vi "MPM_Sample.vi"() -> ()   [LabVIEW 2017]
uses:
  C:/Users/Ssantec_Test/Documents/Instrument_DLL_Sample_Labview_20250826_Ver1.5.0_x64/DLL/InstrumentDLL.dll
  DLL/InstrumentDLL.dll
  <vilib>/Utility/file.llb/Write Delimited Spreadsheet (string).vi
  <vilib>/Utility/file.llb/Write To Spreadsheet File (DBL).vi
panel:
  out "MPM":refnum<k24>
  in  "选项卡控件":T1(tab)
  out "lblver4":string
  out "lblseri4":string
  out "lbltype4":string
  out "lblver3":string
  out "lblseri3":string
  out "lbltype3":string
  out "lblver2":string
  out "lblseri2":string
  out "lbltype2":string
  out "lblver1":string
  out "lblseri1":string
  out "lbltype1":string
  out "lblver0":string
  out "lblseri0":string
  out "lbltype0":string
  out "module count":string
  out "Product":string
  out "Serial":string
  out "F/ W Vesion":string
  in  "btnDisconnect":bool
  in  "btnConnect":bool
  in  "Portnumber":i32
  in  "Address/ComPort":string
  in  "Communication":T2(radio)
  in  "GetComport":bool
  in  "ComPort":u16(ring)
  in  "btnSplit":bool
  out "Address":dbl
  out "Board number":dbl
  in  "btnVisa":bool
  in  "Visa String":u16(ring) items=["GPIB0::16::INSTR"]
  out "txtlan_port":string
  in  "btnGetPort":bool
  out "txtipaddress":string
  in  "btnGetIP":bool
  out "txtsyst_error":string
  in  "btnGetError":bool
  in  "btnGetWavelength":bool
  in  "txtwave_ch":i32 caption="Ch"
  in  "txtwave_slot":i32 caption="Slot"
  in  "btnZeroing":bool
  out "txtreadp_all":string caption="Read Power for each slot"
  in  "txtread_slotall":i32 caption="Slot"
  in  "btnSlot_Power":bool
  out "txt_readp_ch":dbl caption="Read Power for each ch"
  in  "txtread_ch":i32=1 caption="Ch"
  in  "txtread_slot":i32 caption="Slot"
  in  "btnSlot_Ch_Power":bool
  out "txtget_erange":dbl caption="Range for each ch"
  in  "txtget_rangech":i32=1 caption="Ch"
  in  "txtget_rangeslot":i32 caption="Slot"
  out "txtgetrmode":string caption="Range mode for \"READ\""
  in  "btnSlot_Ch_Range":bool
  in  "btnGet":bool
  out "txtget_unit":string caption="Unit"
  out "txtget_avg":dbl caption="Averaging time(msec)"
  out "txtget_wave":dbl caption="Wavelength(nm)"
  out "txtgetrang":i32 caption="Range All"
  in  "Ch":i32
  in  "Slot":i32
  in  "Range for each ch":i32
  in  "btnSetSlot":bool
  in  "Averaging time(msec)":dbl
  in  "btnSetAveraging":bool
  in  "btnSetUnit":bool
  in  "Unit":u16(ring) items=["dBm", "mW"]
  in  "btnSetRangeAll":bool
  in  "Range All":i32
  in  "btnSetRangeMode":bool
  in  "Range mode for \"READ\"":enum16{"Auto", "Manual"}(ring)
  in  "Wavelength(nm)":dbl
  in  "btnSetWavelength":bool
  in  "btnGetSlot":bool
  in  "txte_slot":i32 caption="Slot"
  in  "btnGetch":bool
  in  "txtlog_ch":i32 caption="Ch"
  in  "txtlog_slot":i32 caption="Slot"
  out "txtlog_status":string
  in  "btnStop":bool
  in  "btnStatus":bool
  in  "btnStart":bool
  in  "btnSetFreerun":bool
  in  "cmbfr_tin_mode":enum16{"Internal", "Extarnal"}(ring) caption="Trigger input mode"
  in  "txtfr_range":i32 caption="Range"
  in  "txtfr_point":i32 caption="number of point"
  in  "txtfr_ave":dbl caption="Averaging Time(msec)"
  in  "txtfr_wave":dbl caption="Wavelength(nm)"
  in  "btnSetSweep":bool
  in  "txtsm_range":i32 caption="Range"
  in  "cmbsm_rangemode":enum16{"Auto", "Manual"}(ring) caption="Range mode"
  in  "txtspeed":i32 caption="Speed(nm/sec)"
  in  "txtwavestep":dbl caption="Step wavelenght(nm)"
  in  "txtstopwave":dbl caption="Stop wavelenght(nm)"
  in  "txtstartwave":dbl caption="Start wavelength(nm)"
  in  "txtcon_range":i32 caption="Range"
  in  "cmbcon_rangemode":enum16{"Auto", "Manual"}(ring) caption="Range mode"
  in  "txtcon_point":i32 caption="number of point"
  in  "txtcon_ave":dbl caption="Averaging Time(msec)"
  in  "txtcon_wave":dbl caption="Wavelength(nm)"
  in  "btnSetConst":bool
  in  "btnGetParameter":bool
  out "txtg_speed":dbl caption="Sweep speed(nm)"
  out "txtg_stepwave":dbl caption="Step wavelength(nm)"
  out "txtg_stopwave":dbl caption="Stop wavelength(nm)"
  out "txtg_statwave":dbl caption="Start wavelength(nm)"
  out "txtg_wavelength":dbl caption="Wavelength(nm)"
  out "txtg_settingrange":string caption="Setting Range"
  out "txtg_tinmode":string caption="Trigger input mode"
  out "txtg_rangemode":string caption="Range mode"
  out "txtlog_mode":string caption="SweepMode"
  out "txtg_point":i32 caption="number of point"
  out "txtg_ave":dbl caption="Averaging time"
  # "0. Connect Tool"
  # "1. Connect"
  # "Communication setting"
  # "Information"
  # "Module Information"
  # "Slot0"
  # "Slot1"
  # "Slot2"
  # "Slot3"
  # "Slot4"
  # "Type"
  # "Serial"
  # "Version"
  # "Set"
  # "Get"
  # "Common function"
  # "Const Mode"
  # "Sweep Mode"
  # "FreerunMode"
  # "Common"
  # "Get Parameter"
  # "Sweep mode parameter"
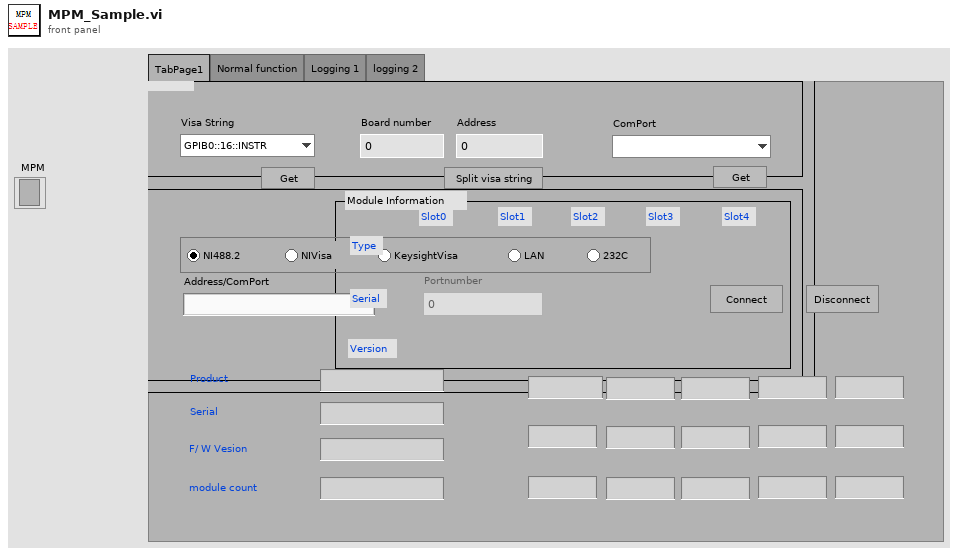
[diagram p1: front panel]
types:
  T1 = enum32{"TabPage1", "Normal function", "Logging 1", "logging 2"}
  T2 = enum32{"rdiNI488", "rdiNIvisa", "rdikeysightvisa", "rdiLAN", "rdi232C"}
  T3 = enum8{"Enabled", "Disabled", "Disabled and Grayed Out"}
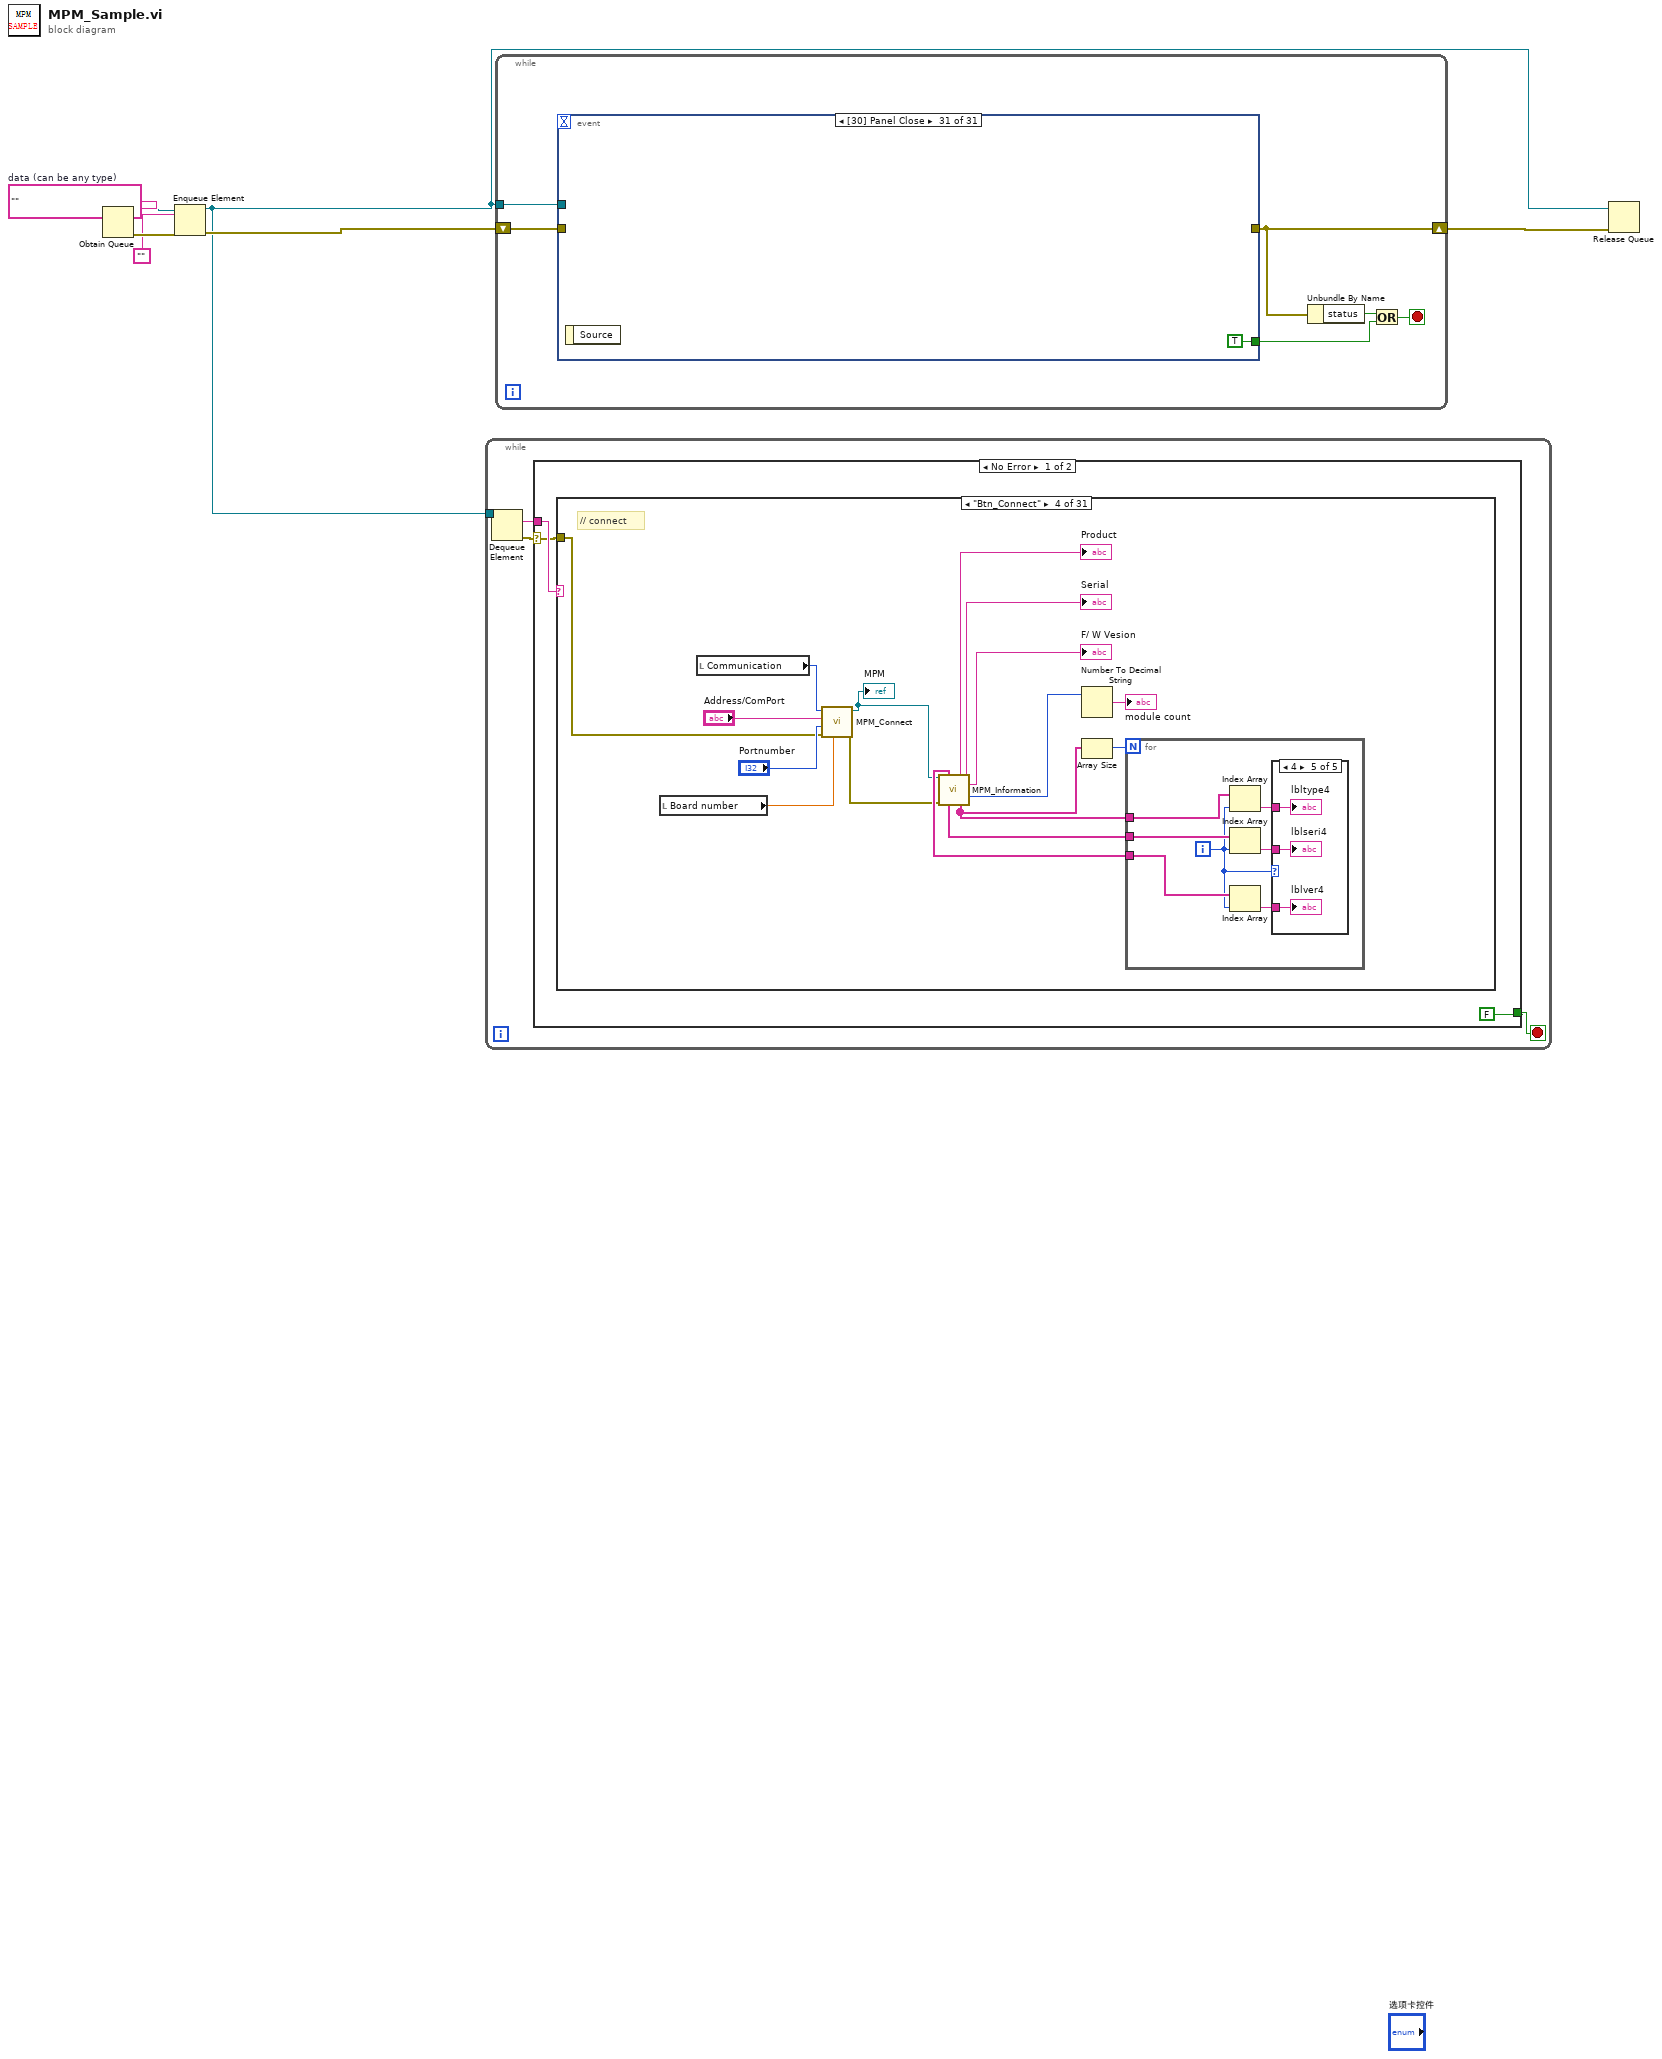
[diagram p0: block diagram]
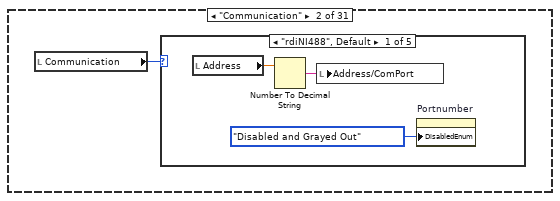
[diagram p3: hidden frame]
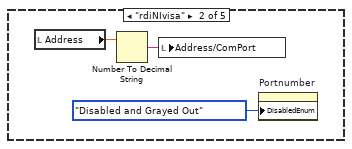
[diagram p4: hidden frame]
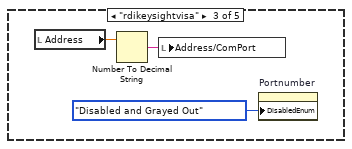
[diagram p5: hidden frame]
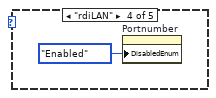
[diagram p6: hidden frame]
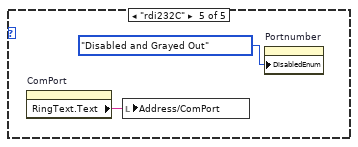
[diagram p7: hidden frame]
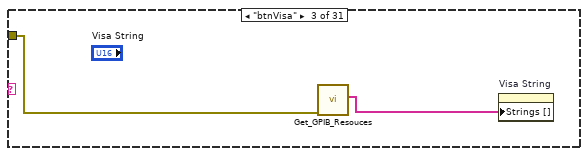
[diagram p8: hidden frame]
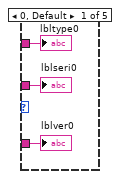
[diagram p9: hidden frame]
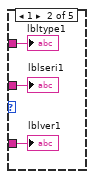
[diagram p10: hidden frame]
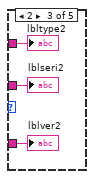
[diagram p11: hidden frame]
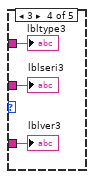
[diagram p12: hidden frame]
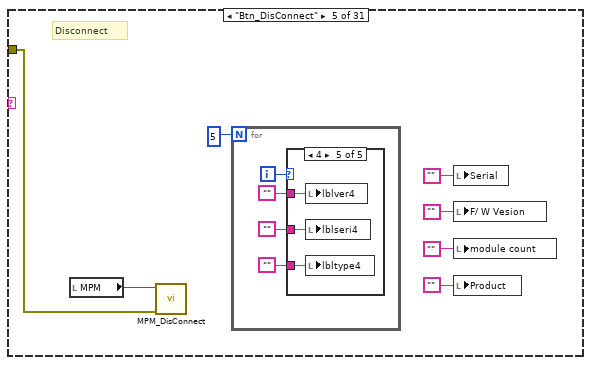
[diagram p13: hidden frame]
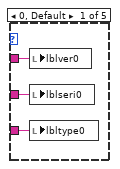
[diagram p14: hidden frame]
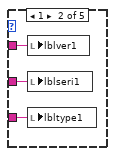
[diagram p15: hidden frame]
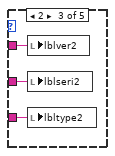
[diagram p16: hidden frame]
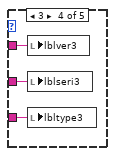
[diagram p17: hidden frame]
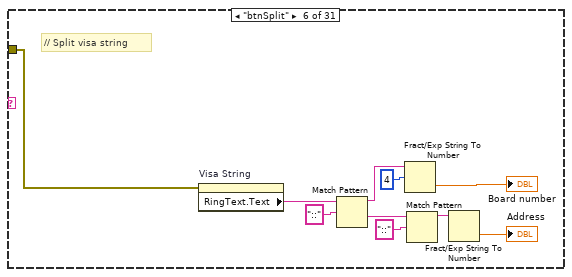
[diagram p18: hidden frame]
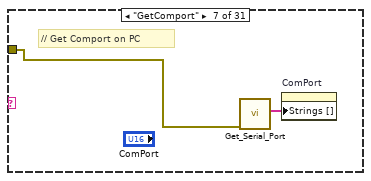
[diagram p19: hidden frame]
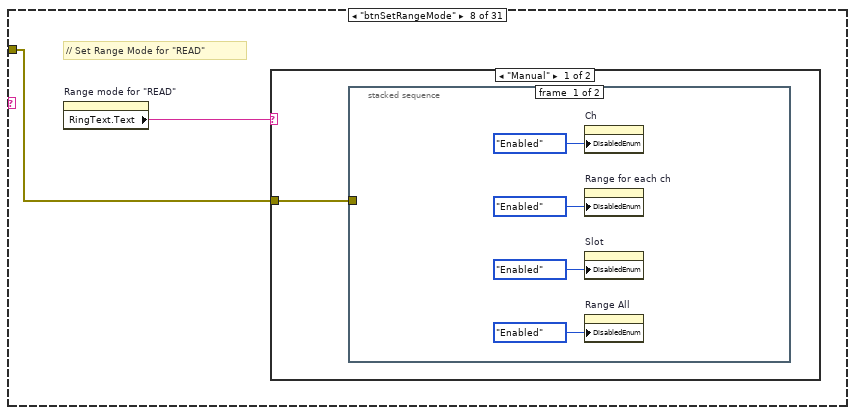
[diagram p20: hidden frame]
diagram:
  w4 = ""  # data (can be any type)
  n1 = Obtain Queue(element data type=w4) -> (queue out=w3:refnum<queue>, error out=w7:errorcluster)  [unwired: 4 in, 1 out]
  n2 = Enqueue Element(queue=w3, element="", error in (no error)=w7) -> (queue out=w1:refnum<queue>, error out=w6:errorcluster)  [unwired: 1 in, 1 out]
  n3 = while {
    tunnel: w1 -> [w11]
    stop <- w8 stop-if-true
    n4 = Dequeue Element(queue=w11) -> (element=w9:string, error out=w10:errorcluster)  [unwired: 2 in, 2 out]
    n5 = case shown="No Error" w10 {
      selector: w10 -> [w12 _]
      tunnel: w9 -> [w13 _]
      tunnel: [FALSE TRUE] -> w8
      frame No Error {
        n6 = case shown="\"Btn_Connect\"" w13 {
          tunnel: w12 -> [_ _ w28 w31 w68 w103 w104 w106 w124 w127 w130 w133 w138 w141 w160 w165 w170 w194 w196 w216 w219 w222 w229 w250 w274 w291 w293 w301 w304 w318 w331]
          frame "Load", Default {
          }
          frame "Communication" {
            n7 = local read "Communication"() -> (w15:T2)
            n8 = case shown="\"rdiNI488\", Default" w15 {
              frame "rdiNI488", Default {
                n9 = local read "Address"() -> (w16:dbl)
                n10 = Number To Decimal String(number=w16) -> (decimal integer string=w17:string)  [unwired: 1 in]
                n11 = local write "Address/ComPort"(w17) -> ()
                n12 = property on="Portnumber" class="DigNum (strict)"("DisabledEnum"=T3."Disabled and Grayed Out" ("禁用")) -> ()  [unwired: 2 in, 2 out]
              }
              frame "rdiNIvisa" {
                n13 = local read "Address"() -> (w19:dbl)
                n14 = Number To Decimal String(number=w19) -> (decimal integer string=w20:string)  [unwired: 1 in]
                n15 = local write "Address/ComPort"(w20) -> ()
                n16 = property on="Portnumber" class="DigNum (strict)"("DisabledEnum"=T3."Disabled and Grayed Out" ("禁用")) -> ()  [unwired: 2 in, 2 out]
              }
              frame "rdikeysightvisa" {
                n17 = local read "Address"() -> (w22:dbl)
                n18 = Number To Decimal String(number=w22) -> (decimal integer string=w23:string)  [unwired: 1 in]
                n19 = local write "Address/ComPort"(w23) -> ()
                n20 = property on="Portnumber" class="DigNum (strict)"("DisabledEnum"=T3."Disabled and Grayed Out" ("禁用")) -> ()  [unwired: 2 in, 2 out]
              }
              frame "rdiLAN" {
                n21 = property on="Portnumber" class="DigNum (strict)"("DisabledEnum"=T3."Enabled" ("禁用")) -> ()  [unwired: 2 in, 2 out]
              }
              frame "rdi232C" {
                n22 = property on="ComPort" class="Ring (strict)"() -> ("RingText.Text"=w26:string)  [unwired: 2 in, 2 out]
                n23 = local write "Address/ComPort"(w26) -> ()
                n24 = property on="Portnumber" class="DigNum (strict)"("DisabledEnum"=T3."Disabled and Grayed Out" ("禁用")) -> ()  [unwired: 2 in, 2 out]
              }
            }
          }
          frame "btnVisa" {
            n25 = call "Get_GPIB_Resouces.vi"("error in (no error)"=w28) -> ("Get_GPIB_Resources"=w29:string[])  [unwired: 8 in, 2 out]
            n26 = property on="Visa String" class="Ring (strict)"("Strings []"=w29) -> ()  [unwired: 2 in, 2 out]
          }
          frame "Btn_Connect" {
            # "// connect"
            n27 = local read "Board number"() -> (w30:dbl)
            n28 = local read "Communication"() -> (w33:T2)
            n29 = call "MPM_Connect.vi"("GPIBBoard"=w30, "error in (no error)"=w31, "Portnumber"="Portnumber", "Address/ComPort"="Address/ComPort", "Communication"=w33) -> ("error out"=w34:errorcluster, "Reference out"=w32:refnum<k24>)  [unwired: 5 in]
            "MPM" <- w32
            n30 = call "MPM_Information.vi"(".NET Reference in"=w32, "error in (no error)"=w34) -> ("ModuleFW"=w38:string[], "ProductName"=→"Product":string, "FWversion"=→"F/ W Vesion":string, "SerialNumber"=→"Serial":string, "NumberofModule"=w44:i32, "ModuelSerial"=w39:string[], "ModuleType"=w36:string[])  [unwired: 5 in, 2 out]
            n31 = Number To Decimal String(number=w44) -> (decimal integer string=→"module count":string)  [unwired: 1 in]
            n32 = Array Size(array=w36) -> (size(s)=w35:i32)
            n33 = for {
              N: w35 -> [_]
              tunnel: w36 -> [w52]
              tunnel: w39 -> [w51]
              tunnel: w38 -> [w50]
              i -> [w49]
              n34 = Index Array(array=w52, index=w49) -> (element=w48:string)
              n35 = Index Array(array=w51, index=w49) -> (element=w47:string)
              n36 = Index Array(array=w50, index=w49) -> (element=w46:string)
              n37 = case shown="4" w49 {
                tunnel: w48 -> [w55 w58 w61 w64 w67]
                tunnel: w47 -> [w54 w57 w60 w63 w66]
                tunnel: w46 -> [w53 w56 w59 w62 w65]
                frame 0, Default {
                  "lbltype0" <- w55
                  "lblseri0" <- w54
                  "lblver0" <- w53
                }
                frame 1 {
                  "lbltype1" <- w58
                  "lblseri1" <- w57
                  "lblver1" <- w56
                }
                frame 2 {
                  "lbltype2" <- w61
                  "lblseri2" <- w60
                  "lblver2" <- w59
                }
                frame 3 {
                  "lbltype3" <- w64
                  "lblseri3" <- w63
                  "lblver3" <- w62
                }
                frame 4 {
                  "lbltype4" <- w67
                  "lblseri4" <- w66
                  "lblver4" <- w65
                }
              }
            }
          }
          frame "Btn_DisConnect" {
            # "Disconnect"
            n38 = local read "MPM"() -> (w74:refnum<k24>)
            n39 = call "MPM_DisConnect.vi"("error in (no error)"=w68, ".NET Reference in"=w74) -> ()  [unwired: 8 in, 2 out]
            n40 = for {
              N: 5 -> [_]
              i -> [w78]
              n41 = case shown="4" w78 {
                tunnel: "" -> [w81 w84 w87 w90 w93]
                tunnel: "" -> [w80 w83 w86 w89 w92]
                tunnel: "" -> [w79 w82 w85 w88 w91]
                frame 0, Default {
                  n42 = local write "lblver0"(w79) -> ()
                  n43 = local write "lblseri0"(w80) -> ()
                  n44 = local write "lbltype0"(w81) -> ()
                }
                frame 1 {
                  n45 = local write "lblver1"(w82) -> ()
                  n46 = local write "lblseri1"(w83) -> ()
                  n47 = local write "lbltype1"(w84) -> ()
                }
                frame 2 {
                  n48 = local write "lblver2"(w85) -> ()
                  n49 = local write "lblseri2"(w86) -> ()
                  n50 = local write "lbltype2"(w87) -> ()
                }
                frame 3 {
                  n51 = local write "lblver3"(w88) -> ()
                  n52 = local write "lblseri3"(w89) -> ()
                  n53 = local write "lbltype3"(w90) -> ()
                }
                frame 4 {
                  n54 = local write "lblver4"(w91) -> ()
                  n55 = local write "lblseri4"(w92) -> ()
                  n56 = local write "lbltype4"(w93) -> ()
                }
              }
            }
            n57 = local write "Serial"("") -> ()
            n58 = local write "F/ W Vesion"("") -> ()
            n59 = local write "module count"("") -> ()
            n60 = local write "Product"("") -> ()
          }
          frame "btnSplit" {
            # "// Split visa string"
            n61 = property on="Visa String" class="Ring (strict)"(error in=w103) -> ("RingText.Text"=w96:string)  [unwired: 1 in, 2 out]
            n62 = Match Pattern(string=w96, regular expression="::") -> (before substring=w99:string, after substring=w100:string)  [unwired: 1 in, 2 out]
            n63 = Fract/Exp String To Number(string=w99, offset=4 ("偏移量")) -> (number=→"Board number":dbl)  [unwired: 2 in, 1 out]
            n64 = Match Pattern(string=w100, regular expression="::") -> (before substring=w97:string)  [unwired: 1 in, 3 out]
            n65 = Fract/Exp String To Number(string=w97) -> (number=→"Address":dbl)  [unwired: 3 in, 1 out]
          }
          frame "GetComport" {
            # "// Get Comport on PC"
            n66 = call "Get_Serial_Port.vi"("error in (no error)"=w104) -> ("Get_Serial_Port"=w105:string[])  [unwired: 8 in, 2 out]
            n67 = property on="ComPort" class="Ring (strict)"("Strings []"=w105) -> ()  [unwired: 2 in, 2 out]
          }
          frame "btnSetRangeMode" {
            # "// Set Range Mode for \"READ\""
            n68 = property on="Range mode for \"READ\"" class="Enum (strict)"() -> ("RingText.Text"=w107:string)  [unwired: 2 in, 2 out]
            n69 = case shown="\"Manual\"" w107 {
              tunnel: w106 -> [w108 w116]
              frame "Manual" {
                n70 = stacked-sequence {
                  tunnel: w108 -> [_ w113]
                  frame #0 {
                    n71 = property on="Ch" class="DigNum (strict)"("DisabledEnum"=T3."Enabled" ("禁用")) -> ()  [unwired: 2 in, 2 out]
                    n72 = property on="Range for each ch" class="DigNum (strict)"("DisabledEnum"=T3."Enabled" ("禁用")) -> ()  [unwired: 2 in, 2 out]
                    n73 = property on="Slot" class="DigNum (strict)"("DisabledEnum"=T3."Enabled" ("禁用")) -> ()  [unwired: 2 in, 2 out]
                    n74 = property on="Range All" class="DigNum (strict)"("DisabledEnum"=T3."Enabled" ("禁用")) -> ()  [unwired: 2 in, 2 out]
                  }
                  frame #1 {
                    n75 = local read "Range mode for \"READ\""() -> (w115:enum16{"Auto", "Manual"})
                    n76 = local read "MPM"() -> (w114:refnum<k24>)
                    n77 = call "MPM_Set_Read_Rang_Mode.vi"("error in (no error)"=w113, "mode"=w115, ".NET Reference in"=w114) -> ()  [unwired: 7 in, 2 out]
                  }
                }
              }
              frame "Auto", Default {
                n78 = stacked-sequence {
                  tunnel: w116 -> [_ w121]
                  frame #0 {
                    n79 = property on="Slot" class="DigNum (strict)"("DisabledEnum"=T3."Disabled" ("禁用")) -> ()  [unwired: 2 in, 2 out]
                    n80 = property on="Range for each ch" class="DigNum (strict)"("DisabledEnum"=T3."Disabled" ("禁用")) -> ()  [unwired: 2 in, 2 out]
                    n81 = property on="Range All" class="DigNum (strict)"("DisabledEnum"=T3."Disabled" ("禁用")) -> ()  [unwired: 2 in, 2 out]
                    n82 = property on="Ch" class="DigNum (strict)"("DisabledEnum"=T3."Disabled" ("禁用")) -> ()  [unwired: 2 in, 2 out]
                  }
                  frame #1 {
                    n83 = local read "MPM"() -> (w123:refnum<k24>)
                    n84 = call "MPM_Set_Read_Rang_Mode.vi"("error in (no error)"=w121, "mode"="Range mode for \"READ\"", ".NET Reference in"=w123) -> ()  [unwired: 7 in, 2 out]
                  }
                }
              }
            }
          }
          frame "btnSetRangeAll" {
            # "// Set range for munal range\n            // MPM-211/212 : 1～5 MPM213 : 1～4　　MPM215 : Nothing"
            n85 = local read "MPM"() -> (w126:refnum<k24>)
            n86 = call "MPM_Set_Range.vi"("error in (no error)"=w124, "Range All"="Range All", ".NET Reference in"=w126) -> ()  [unwired: 7 in, 2 out]
          }
          frame "btnSetWavelength" {
            # "// Set Wavelength(nm)"
            n87 = local read "MPM"() -> (w129:refnum<k24>)
            n88 = call "MPM_Set_Wavelength.vi"("error in (no error)"=w127, "Wavelength(nm)"="Wavelength(nm)", ".NET Reference in"=w129) -> ()  [unwired: 7 in, 2 out]
          }
          frame "btnSetUnit" {
            # "// Set Power unit"
            n89 = local read "MPM"() -> (w132:refnum<k24>)
            n90 = call "MPM_Set_Unit.vi"("error in (no error)"=w130, "unit"="Unit", ".NET Reference in"=w132) -> ()  [unwired: 7 in, 2 out]
          }
          frame "btnSetAveraging" {
            # "// Set Averaging Time(mse)\n            // MPM can set 0.01msec～10000msec"
            n91 = local read "MPM"() -> (w135:refnum<k24>)
            n92 = call "MPM_Set_Averaging_Time.vi"("error in (no error)"=w133, "Averaging time(msec)"="Averaging time(msec)", ".NET Reference in"=w135) -> ()  [unwired: 7 in, 2 out]
          }
          frame "btnSetSlot" {
            # "// Set Range for each ch"
            n93 = local read "MPM"() -> (w140:refnum<k24>)
            n94 = call "MPM_Set_Range_Each_Channel.vi"("Range for each ch"="Range for each ch", "error in (no error)"=w138, "Ch"="Ch", "Slot"="Slot", ".NET Reference in"=w140) -> ()  [unwired: 5 in, 2 out]
          }
          frame "btnGet" {
            # "// Get normal function parameter"
            n95 = local read "MPM"() -> (w155:refnum<k24>)
            n96 = call "MPM_Get_Read_Range_Mode.vi"("error in (no error)"=w141, ".NET Reference in"=w155) -> ("error out"=w153:errorcluster, "mode"=w142:enum16{"Manual", "Auto"}, "Reference out"=w154:refnum<k24>)  [unwired: 7 in]
            n97 = case shown="\"Auto\"" w142 {
              frame "Manual", Default {
                n98 = local write "txtgetrmode"("Manual") -> ()
              }
              frame "Auto" {
                "txtgetrmode" <- "Auto"
              }
            }
            n99 = call "MPM_Get_Range.vi"("error in (no error)"=w153, ".NET Reference in"=w154) -> ("error out"=w151:errorcluster, "range out"=→"txtgetrang":i32, "Reference out"=w152:refnum<k24>)  [unwired: 7 in]
            n100 = call "MPM_Get_Wavelength.vi"("error in (no error)"=w151, ".NET Reference in"=w152) -> ("error out"=w148:errorcluster, "wave out"=→"txtget_wave":dbl, "Reference out"=w149:refnum<k24>)  [unwired: 7 in]
            n101 = call "MPM_Get_Averaging_Time.vi"("error in (no error)"=w148, ".NET Reference in"=w149) -> ("error out"=w145:errorcluster, "time out"=→"txtget_avg":dbl, "Reference out"=w146:refnum<k24>)  [unwired: 7 in]
            n102 = call "MPM_Get_Unit.vi"("error in (no error)"=w145, ".NET Reference in"=w146) -> ("unit"=w143:enum16{"dBmA, dBm", "mW, mA"})  [unwired: 7 in, 2 out]
            n103 = case shown="\"mW, mA\"" w143 {
              frame "dBmA, dBm", Default {
                n104 = local write "txtget_unit"("dBm") -> ()
              }
              frame "mW, mA" {
                "txtget_unit" <- "mW"
              }
            }
          }
          frame "btnSlot_Ch_Range" {
            # "// Get Range for each ch"
            n105 = local read "MPM"() -> (w164:refnum<k24>)
            n106 = call "MPM_Get_Range_Each_for_Channel.vi"("error in (no error)"=w160, "channelNumber"="txtget_rangech", "moduleNumber"="txtget_rangeslot", ".NET Reference in"=w164) -> ("range out"=→"txtget_erange":i32)  [unwired: 5 in, 2 out]
          }
          frame "btnSlot_Ch_Power" {
            # "// Read Power for each ch"
            n107 = local read "MPM"() -> (w169:refnum<k24>)
            n108 = call "MPM_Get_READ_Power_for_Channel.vi"("error in (no error)"=w165, "channelNumber"="txtread_ch", "moduleNumber"="txtread_slot", ".NET Reference in"=w169) -> ("power out"=→"txt_readp_ch":dbl)  [unwired: 5 in, 2 out]
          }
          frame "btnSlot_Power" {
            # "// Read Power for Slot"
            n109 = local read "MPM"() -> (w193:refnum<k24>)
            n110 = call "MPM_Get_READ_Power_for_Module.vi"("error in (no error)"=w170, "moduleNumber"="txtread_slotall", ".NET Reference in"=w193) -> ("powers out"=w175:dbl[])  [unwired: 6 in, 2 out]
            n111 = Index Array(array=w175, index #1=0 ("索引"), index #2=1 ("索引"), index #3=2 ("索引"), index #4=3 ("索引")) -> (element #1=w184:dbl, element #2=w185:dbl, element #3=w186:dbl, element #4=w187:dbl)
            n112 = Number To Fractional String(number=w184, precision (6)=i16 3 ("精度(6)")) -> (F-format string=w182:string)  [unwired: 2 in]
            n113 = Number To Fractional String(number=w185, precision (6)=i16 3 ("精度(6)")) -> (F-format string=w180:string)  [unwired: 2 in]
            n114 = Number To Fractional String(number=w186, precision (6)=i16 3 ("精度(6)")) -> (F-format string=w178:string)  [unwired: 2 in]
            n115 = Number To Fractional String(number=w187, precision (6)=i16 3 ("精度(6)")) -> (F-format string=w176:string)  [unwired: 2 in]
            n116 = Concatenate Strings(w182, "," ("字符串"), w180, "," ("字符串"), w178, "," ("字符串"), w176) -> (→"txtreadp_all":string)
          }
          frame "btnZeroing" {
            # "// Zeroing function"
            n117 = local read "MPM"() -> (w195:refnum<k24>)
            n118 = call "MPM_Zeroing.vi"("error in (no error)"=w194, ".NET Reference in"=w195) -> ()  [unwired: 8 in, 2 out]
          }
          frame "btnGetWavelength" {
            # "// Get Wavelength Sencitvity data for each ch"
            n119 = local read "MPM"() -> (w205:refnum<k24>)
            n120 = call "MPM_Get_Wavelength_Senctivity_Data.vi"("error in (no error)"=w196, "channelNumber"="txtwave_ch", "moduleNumber"="txtwave_slot", ".NET Reference in"=w205) -> ("offsetpower out"=w199:sgl[], "wavedata out"=w198:dbl[])  [unwired: 4 in, 2 out]
            n121 = Array Size(array=w198) -> (size(s)=w203:i32)
            n122 = for {
              N: w203 -> [_]
              tunnel: w199 -> [w215]
              tunnel: w198 -> [w214]
              tunnel: [w206] -> w202
              i -> [w213]
              n123 = Index Array(array=w214, index=w213) -> (element=w212:dbl)
              n124 = Index Array(array=w215, index=w213) -> (element=w211:sgl)
              n125 = Number To Hexadecimal String(2:w212) -> (0:w210:string)  [unwired: 1 in]
              n126 = Number To Hexadecimal String(2:w211) -> (0:w209:string)  [unwired: 1 in]
              n127 = Concatenate Strings(w210, "，" ("字符串"), w209) -> (w207:string)
              n128 = Initialize Array(w207) -> (w206:string[])  [unwired: 1 in]
            }
            n129 = call-poly <vilib>:"Write Delimited Spreadsheet.vi"("format (%s)"="%s", "1D data"=w202, "transpose? (no:F)"=FALSE ("transpose? (F)")) -> ()  [unwired: 11 in, 2 out]
          }
          frame "btnGetError" {
            # "// Get MPM error code"
            n130 = local read "MPM"() -> (w218:refnum<k24>)
            n131 = call "MPM_Get_System_Error.vi"("error in (no error)"=w216, ".NET Reference in"=w218) -> ("error"=→"txtsyst_error":string)  [unwired: 7 in, 2 out]
          }
          frame "btnGetIP" {
            n132 = local read "MPM"() -> (w221:refnum<k24>)
            n133 = call "MPM_Get_IPAddress.vi"("error in (no error)"=w219, ".NET Reference in"=w221) -> ("address out"=→"txtipaddress":string)  [unwired: 7 in, 2 out]
          }
          frame "btnGetPort" {
            n134 = local read "MPM"() -> (w225:refnum<k24>)
            n135 = call "MPM_Get_LAN_PortNumber.vi"("error in (no error)"=w222, ".NET Reference in"=w225) -> ("port out"=w223:i32)  [unwired: 7 in, 2 out]
            n136 = Number To Decimal String(number=w223) -> (decimal integer string=→"txtlan_port":string)  [unwired: 1 in]
          }
          frame "btnSetConst" {
            w234 = 1 items=["Internal", "Extarnal"] ("mode")
            n137 = local read "MPM"() -> (w227:refnum<k24>)
            n138 = call "MPM_Set_Averaging_Time.vi"("error in (no error)"=w229, "Averaging time(msec)"="txtcon_ave", ".NET Reference in"=w227) -> ("error out"=w232:errorcluster, "Reference out"=w237:refnum<k24>)  [unwired: 7 in]
            n139 = call "MPM_Set_Logging_Data_Point.vi"("error in (no error)"=w232, "count"="txtcon_point", ".NET Reference in"=w237) -> ("error out"=w231:errorcluster, "Reference out"=w236:refnum<k24>)  [unwired: 7 in]
            n140 = call "MPM_Set_Wavelength.vi"("error in (no error)"=w231, "Wavelength(nm)"="txtcon_wave", ".NET Reference in"=w236) -> ("error out"=w230:errorcluster, "Reference out"=w233:refnum<k24>)  [unwired: 7 in]
            n141 = call "MPM_Set_Trigger_Input_Mode.vi"("error in (no error)"=w230, "mode"=w234, ".NET Reference in"=w233) -> ("error out"=w228:errorcluster, "Reference out"=w226:refnum<k24>)  [unwired: 7 in]
            n142 = case shown="\"Auto\", Default" "cmbcon_rangemode" {
              tunnel: w226 -> [w242 w249]
              tunnel: w228 -> [w241 w244]
              frame "Auto", Default {
                w243 = 2 items=["ManualRangeConstant", "ManualRangeSweep", "AutoRangeConstant", "AutoRangeSweep", "Freerun"] ("mode")
                n143 = call "MPM_Set_Mode.vi"("error in (no error)"=w241, "mode"=w243, ".NET Reference in"=w242) -> ()  [unwired: 7 in, 2 out]
              }
              frame "Manual" {
                w248 = 0 items=["ManualRangeConstant", "ManualRangeSweep", "AutoRangeConstant", "AutoRangeSweep", "Freerun"] ("mode")
                n144 = call "MPM_Set_Mode.vi"("error in (no error)"=w244, "mode"=w248, ".NET Reference in"=w249) -> ("error out"=w245:errorcluster, "Reference out"=w246:refnum<k24>)  [unwired: 7 in]
                n145 = call "MPM_Set_Range.vi"("error in (no error)"=w245, "Range All"="txtcon_range", ".NET Reference in"=w246) -> ()  [unwired: 7 in, 2 out]
              }
            }
          }
          frame "btnSetSweep" {
            w254 = 1 items=["Internal", "Extarnal"] ("mode")
            n146 = local read "MPM"() -> (w253:refnum<k24>)
            n147 = call "MPM_Set_Trigger_Input_Mode.vi"("error in (no error)"=w250, "mode"=w254, ".NET Reference in"=w253) -> ("error out"=w255:errorcluster, "Reference out"=w256:refnum<k24>)  [unwired: 7 in]
            n148 = call "MPM_Set_Sweep_Wavelength.vi"("wavestep"="txtwavestep", "error in (no error)"=w255, "stopwave"="txtstopwave", "startwave"="txtstartwave", ".NET Reference in"=w256) -> ("error out"=w259:errorcluster, "Reference out"=w260:refnum<k24>)  [unwired: 5 in]
            n149 = call "MPM_Set_Sweep_Speed.vi"("error in (no error)"=w259, "speed"="txtspeed", ".NET Reference in"=w260) -> ("error out"=w251:errorcluster, "Reference out"=w252:refnum<k24>)  [unwired: 7 in]
            n150 = case shown="\"Auto\", Default" "cmbsm_rangemode" {
              tunnel: w252 -> [w265 w271]
              tunnel: w251 -> [w264 w267]
              frame "Auto", Default {
                w266 = 3 items=["ManualRangeConstant", "ManualRangeSweep", "AutoRangeConstant", "AutoRangeSweep", "Freerun"] ("mode")
                n151 = call "MPM_Set_Mode.vi"("error in (no error)"=w264, "mode"=w266, ".NET Reference in"=w265) -> ()  [unwired: 7 in, 2 out]
              }
              frame "Manual" {
                w272 = 1 items=["ManualRangeConstant", "ManualRangeSweep", "AutoRangeConstant", "AutoRangeSweep", "Freerun"] ("mode")
                n152 = call "MPM_Set_Mode.vi"("error in (no error)"=w267, "mode"=w272, ".NET Reference in"=w271) -> ("error out"=w268:errorcluster, "Reference out"=w269:refnum<k24>)  [unwired: 7 in]
                n153 = call "MPM_Set_Range.vi"("error in (no error)"=w268, "Range All"="txtsm_range", ".NET Reference in"=w269) -> ()  [unwired: 7 in, 2 out]
              }
            }
          }
          frame "btnSetFreerun" {
            w289 = 4 items=["ManualRangeConstant", "ManualRangeSweep", "AutoRangeConstant", "AutoRangeSweep", "Freerun"] ("mode")
            n154 = local read "MPM"() -> (w290:refnum<k24>)
            n155 = call "MPM_Set_Mode.vi"("error in (no error)"=w274, "mode"=w289, ".NET Reference in"=w290) -> ("error out"=w278:errorcluster, "Reference out"=w288:refnum<k24>)  [unwired: 7 in]
            n156 = call "MPM_Set_Range.vi"("error in (no error)"=w278, "Range All"="txtfr_range", ".NET Reference in"=w288) -> ("error out"=w277:errorcluster, "Reference out"=w286:refnum<k24>)  [unwired: 7 in]
            n157 = call "MPM_Set_Averaging_Time.vi"("error in (no error)"=w277, "Averaging time(msec)"="txtfr_ave", ".NET Reference in"=w286) -> ("error out"=w279:errorcluster, "Reference out"=w284:refnum<k24>)  [unwired: 7 in]
            n158 = call "MPM_Set_Logging_Data_Point.vi"("error in (no error)"=w279, "count"="txtfr_point", ".NET Reference in"=w284) -> ("error out"=w276:errorcluster, "Reference out"=w281:refnum<k24>)  [unwired: 7 in]
            n159 = call "MPM_Set_Wavelength.vi"("error in (no error)"=w276, "Wavelength(nm)"="txtfr_wave", ".NET Reference in"=w281) -> ("error out"=w275:errorcluster, "Reference out"=w280:refnum<k24>)  [unwired: 7 in]
            n160 = call "MPM_Set_Trigger_Input_Mode.vi"("error in (no error)"=w275, "mode"="cmbfr_tin_mode", ".NET Reference in"=w280) -> ()  [unwired: 7 in, 2 out]
          }
          frame "btnStart" {
            n161 = local read "MPM"() -> (w292:refnum<k24>)
            n162 = call "MPM_Logging_Start.vi"("error in (no error)"=w291, ".NET Reference in"=w292) -> ()  [unwired: 8 in, 2 out]
          }
          frame "btnStatus" {
            n163 = local read "MPM"() -> (w300:refnum<k24>)
            n164 = call "MPM_Get_Logging_Status.vi"("error in (no error)"=w293, ".NET Reference in"=w300) -> ("count out"=w295:i32, "status out"=w294:i32)  [unwired: 6 in, 2 out]
            n165 = Number To Decimal String(number=w294) -> (decimal integer string=w298:string)  [unwired: 1 in]
            n166 = Number To Decimal String(number=w295) -> (decimal integer string=w297:string)  [unwired: 1 in]
            n167 = Concatenate Strings(w298, "," ("字符串"), w297) -> (→"txtlog_status":string)
          }
          frame "btnStop" {
            n168 = local read "MPM"() -> (w302:refnum<k24>)
            n169 = call "MPM_Logging_Stop.vi"("error in (no error)"=w301, ".NET Reference in"=w302) -> ()  [unwired: 8 in, 2 out]
          }
          frame "btnGetch" {
            n170 = local read "MPM"() -> (w308:refnum<k24>)
            n171 = call "MPM_Get_Each_Channel_Logdata.vi"("error in (no error)"=w304, "channelNumber"="txtlog_ch", "moduleNumber"="txtlog_slot", ".NET Reference in"=w308) -> ("data out"=w303:sgl[])  [unwired: 5 in, 2 out]
            n172 = call-poly <vilib>:"Write To Spreadsheet File.vi"("transpose? (no:F)"=TRUE, "1D data"=w303) -> ()  [unwired: 6 in, 1 out]
          }
          frame "btnGetSlot" {
            n173 = local read "MPM"() -> (w323:refnum<k24>)
            n174 = call "MPM_Get_Each_Module_Loggdata.vi"("error in (no error)"=w318, "moduleNumber"="txte_slot", ".NET Reference in"=w323) -> ("data out"=w316:sgl[][])  [unwired: 6 in, 2 out]
            n175 = Array Size(array=w316) -> (size(s)=w320:i32[])
            n176 = Index Array(array=w320, index=0 ("索引")) -> (element=w314:i32)
            n177 = Number To Fractional String ("数値を小数文字列に変換")(number=w316, precision (6)=i16 6 ("精度(6)")) -> (F-format string=w313:string[][])  [unwired: 2 in]
            n178 = for {
              N: w314 -> [_]
              shift-right: [w324] -> w317
              shift-left: string[] [] -> [w326]
              i -> [w330]
              n179 = Increment(x=w330) -> (x+1=w329:i32)
              n180 = Format Into String(format string="%d", initial string="Ch", w329) -> (resulting string=w325:string)  [unwired: 1 in, 1 out]
              n181 = Build Array (concatenate)(w326, w325) -> (w324:string[])
            }
            n182 = Transpose 2D Array(2D array=w313) -> (transposed array=w312:string[][])
            n183 = Build Array (concatenate)(w317, w312) -> (w311:string[][])
            n184 = call-poly <vilib>:"Write Delimited Spreadsheet.vi"("format (%s)"="%s", "2D data"=w311, "delimiter (\\t)"="," ("delimiter (\\t)")) -> ()  [unwired: 11 in, 2 out]
          }
          frame "btnGetParameter" {
            n185 = stacked-sequence {
              tunnel: w331 -> [w332 w359]
              frame #0 {
                n186 = local read "MPM"() -> (w346:refnum<k24>)
                n187 = call "MPM_Get_Mode.vi"("error in (no error)"=w332, ".NET Reference in"=w346) -> ("error out"=w343:errorcluster, "mode"=w345:i32, "Reference out"=w344:refnum<k24>)  [unwired: 7 in]
                n188 = case shown="0, Default" w345 {
                  frame 0, Default {
                    "txtg_rangemode" <- "Manual"
                    "txtlog_mode" <- "Const1"
                  }
                  frame 1 {
                    n189 = local write "txtg_rangemode"("Manual") -> ()
                    n190 = local write "txtlog_mode"("Sweep1") -> ()
                  }
                  frame 2 {
                    n191 = local write "txtg_rangemode"("Auto") -> ()
                    n192 = local write "txtlog_mode"("Const2") -> ()
                  }
                  frame 3 {
                    n193 = local write "txtg_rangemode"("Auto") -> ()
                    n194 = local write "txtlog_mode"("Sweep2") -> ()
                  }
                  frame 4 {
                    n195 = local write "txtg_rangemode"("Manual") -> ()
                    n196 = local write "txtlog_mode"("Freerun") -> ()
                  }
                }
                n197 = call "MPM_Get_Averaging_Time.vi"("error in (no error)"=w343, ".NET Reference in"=w344) -> ("error out"=w335:errorcluster, "time out"=→"txtg_ave":dbl, "Reference out"=w336:refnum<k24>)  [unwired: 7 in]
                n198 = call "MPM_Get_Logging_Data_Point.vi"("error in (no error)"=w335, ".NET Reference in"=w336) -> ("error out"=w333:errorcluster, "count out"=→"txtg_point":i32, "Reference out"=w334:refnum<k24>)  [unwired: 7 in]
                n199 = call "MPM_Get_Wavelength.vi"("error in (no error)"=w333, ".NET Reference in"=w334) -> ("error out"=w338:errorcluster, "wave out"=→"txtg_wavelength":dbl, "Reference out"=w339:refnum<k24>)  [unwired: 7 in]
                n200 = call "MPM_Get_Trigger_Input_Mode.vi"("error in (no error)"=w338, ".NET Reference in"=w339) -> ("mode"=w340:i32)  [unwired: 7 in, 2 out]
                n201 = case shown="1" w340 {
                  frame 0, Default {
                    "txtg_tinmode" <- "Internal"
                  }
                  frame 1 {
                    n202 = local write "txtg_tinmode"("Extarnal") -> ()
                  }
                }
              }
              frame #1 {
                n203 = local read "txtg_rangemode"() -> (w362:string)
                n204 = local read "txtlog_mode"() -> (w363:string)
                n205 = Equal?(x=w362, y="Manual") -> (x = y?=w360:bool)
                n206 = Match Pattern(string=w363, regular expression="Sweep") -> (offset past match=w365:i32)  [unwired: 1 in, 3 out]
                n207 = case shown="True" w360 {
                  tunnel: w359 -> [_ w369]
                  frame False {
                    "txtg_settingrange" <- ""
                  }
                  frame True {
                    n208 = local read "MPM"() -> (w371:refnum<k24>)
                    n209 = call "MPM_Get_Range.vi"("error in (no error)"=w369, ".NET Reference in"=w371) -> ("range out"=w370:i32)  [unwired: 7 in, 2 out]
                    n210 = Number To Decimal String(number=w370) -> (decimal integer string=w372:string)  [unwired: 1 in]
                    n211 = local write "txtg_settingrange"(w372) -> ()
                  }
                }
                n212 = Not Equal?(x=w365, y=-1) -> (x != y?=w367:bool)
                n213 = case shown="False" w367 {
                  tunnel: w359 -> [w373 _]
                  frame False {
                    n214 = local read "MPM"() -> (w380:refnum<k24>)
                    n215 = call "MPM_Get_Sweep_Wavelength.vi"("error in (no error)"=w373, ".NET Reference in"=w380) -> ("error out"=w375:errorcluster, "stopwave out"=→"txtg_stopwave":dbl, "startwave out"=→"txtg_statwave":dbl, "Reference out"=w376:refnum<k24>, "stepwave out"=→"txtg_stepwave":dbl)  [unwired: 5 in]
                    n216 = call "MPM_Get_Sweep_Speed.vi"("error in (no error)"=w375, ".NET Reference in"=w376) -> ("speed"=→"txtg_speed":dbl)  [unwired: 7 in, 2 out]
                  }
                  frame True {
                    n217 = Decimal String To Number(string="") -> (number=w382:i32)  [unwired: 2 in, 1 out]
                    n218 = local write "txtg_ave"(w382) -> ()
                  }
                }
              }
            }
          }
        }
      }
      frame Error {
      }
    }
  }
  n219 = while {
    tunnel: w1 -> [w384]
    shift-right: [w386] -> w5
    shift-left: w6 -> [w385]
    stop <- w387 stop-if-true
    n220 = event shown="[30] Panel Close" {
      selector: _ -> [_ _ _ _ _ _ _ _ _ _ _ _ _ _ _ _ _ _ _ _ _ _ _ _ _ _ _ _ _ _ _]
      dyn-events: _ -> [_ _ _ _ _ _ _ _ _ _ _ _ _ _ _ _ _ _ _ _ _ _ _ _ _ _ _ _ _ _ _]
      timeout: _ -> [_ _ _ _ _ _ _ _ _ _ _ _ _ _ _ _ _ _ _ _ _ _ _ _ _ _ _ _ _ _ _]
      tunnel: w385 -> [w393 w395 w400 w405 w409 w411 w416 w419 w423 w427 w431 w435 w439 w443 w447 w451 w455 w459 w463 w467 w471 w475 w479 w483 w487 w491 w495 w499 w503 w507 _]
      tunnel: [w392 w397 w399 w403 w407 w413 w415 w421 w425 w429 w433 w437 w441 w445 w449 w453 w457 w461 w465 w469 w473 w477 w481 w485 w489 w493 w497 w501 w505 w509 _] -> w386
      tunnel: [FALSE ("stop") _ _ _ _ _ _ _ _ _ _ _ _ _ _ _ _ _ _ _ _ _ _ _ _ _ _ _ _ _ TRUE ("stop")] -> w388
      tunnel: w384 -> [w394 w396 w401 w404 w408 w412 w417 w420 w424 w428 w432 w436 w440 w444 w448 w452 w456 w460 w464 w468 w472 w476 w480 w484 w488 w492 w496 w500 w504 w508 _]
      event "btnConnect": Value Change {
        n221 = event-data() -> ()  [unwired: 1 in, 1 out]
        n222 = Enqueue Element(queue=w394, element="Btn_Connect" ("元素"), error in (no error)=w393) -> (error out=w392:errorcluster)  [unwired: 1 in, 2 out]
      }
      event "btnDisconnect": Value Change {
        n223 = event-data() -> ()  [unwired: 1 in, 1 out]
        n224 = Enqueue Element(queue=w396, element="Btn_DisConnect" ("元素"), error in (no error)=w395) -> (error out=w397:errorcluster)  [unwired: 1 in, 2 out]
      }
      event "btnSplit": Value Change {
        n225 = event-data() -> ()  [unwired: 1 in, 1 out]
        n226 = Enqueue Element(queue=w401, element="btnSplit" ("元素"), error in (no error)=w400) -> (error out=w399:errorcluster)  [unwired: 1 in, 2 out]
      }
      event "GetComport": Value Change {
        n227 = event-data() -> ()  [unwired: 1 in, 1 out]
        n228 = Enqueue Element(queue=w404, element="GetComport" ("元素"), error in (no error)=w405) -> (error out=w403:errorcluster)  [unwired: 1 in, 2 out]
      }
      event "btnSetRangeMode": Value Change {
        n229 = event-data() -> ()  [unwired: 1 in, 1 out]
        n230 = Enqueue Element(queue=w408, element="btnSetRangeMode" ("元素"), error in (no error)=w409) -> (error out=w407:errorcluster)  [unwired: 1 in, 2 out]
      }
      event "btnSetRangeAll": Value Change {
        n231 = event-data() -> ()  [unwired: 1 in, 1 out]
        n232 = Enqueue Element(queue=w412, element="btnSetRangeAll" ("元素"), error in (no error)=w411) -> (error out=w413:errorcluster)  [unwired: 1 in, 2 out]
      }
      event "btnSetWavelength": Value Change {
        n233 = event-data() -> ()  [unwired: 1 in, 1 out]
        n234 = Enqueue Element(queue=w417, element="btnSetWavelength" ("元素"), error in (no error)=w416) -> (error out=w415:errorcluster)  [unwired: 1 in, 2 out]
      }
      event "btnSetUnit": Value Change {
        n235 = event-data() -> ()  [unwired: 1 in, 1 out]
        n236 = Enqueue Element(queue=w420, element="btnSetUnit" ("元素"), error in (no error)=w419) -> (error out=w421:errorcluster)  [unwired: 1 in, 2 out]
      }
      event "btnSetAveraging": Value Change {
        n237 = event-data() -> ()  [unwired: 1 in, 1 out]
        n238 = Enqueue Element(queue=w424, element="btnSetAveraging" ("元素"), error in (no error)=w423) -> (error out=w425:errorcluster)  [unwired: 1 in, 2 out]
      }
      event "btnSetSlot": Value Change {
        n239 = event-data() -> ()  [unwired: 1 in, 1 out]
        n240 = Enqueue Element(queue=w428, element="btnSetSlot" ("元素"), error in (no error)=w427) -> (error out=w429:errorcluster)  [unwired: 1 in, 2 out]
      }
      event "btnGet": Value Change {
        n241 = event-data() -> ()  [unwired: 1 in, 1 out]
        n242 = Enqueue Element(queue=w432, element="btnGet" ("元素"), error in (no error)=w431) -> (error out=w433:errorcluster)  [unwired: 1 in, 2 out]
      }
      event "btnSlot_Ch_Range": Value Change {
        n243 = event-data() -> ()  [unwired: 1 in, 1 out]
        n244 = Enqueue Element(queue=w436, element="btnSlot_Ch_Range" ("元素"), error in (no error)=w435) -> (error out=w437:errorcluster)  [unwired: 1 in, 2 out]
      }
      event "btnSlot_Ch_Power": Value Change {
        n245 = event-data() -> ()  [unwired: 1 in, 1 out]
        n246 = Enqueue Element(queue=w440, element="btnSlot_Ch_Power" ("元素"), error in (no error)=w439) -> (error out=w441:errorcluster)  [unwired: 1 in, 2 out]
      }
      event "btnSlot_Power": Value Change {
        n247 = event-data() -> ()  [unwired: 1 in, 1 out]
        n248 = Enqueue Element(queue=w444, element="btnSlot_Power" ("元素"), error in (no error)=w443) -> (error out=w445:errorcluster)  [unwired: 1 in, 2 out]
      }
      event "btnZeroing": Value Change {
        n249 = event-data() -> ()  [unwired: 1 in, 1 out]
        n250 = Enqueue Element(queue=w448, element="btnZeroing" ("元素"), error in (no error)=w447) -> (error out=w449:errorcluster)  [unwired: 1 in, 2 out]
      }
      event "btnGetWavelength": Value Change {
        n251 = event-data() -> ()  [unwired: 1 in, 1 out]
        n252 = Enqueue Element(queue=w452, element="btnGetWavelength" ("元素"), error in (no error)=w451) -> (error out=w453:errorcluster)  [unwired: 1 in, 2 out]
      }
      event "btnGetError": Value Change {
        n253 = event-data() -> ()  [unwired: 1 in, 1 out]
        n254 = Enqueue Element(queue=w456, element="btnGetError" ("元素"), error in (no error)=w455) -> (error out=w457:errorcluster)  [unwired: 1 in, 2 out]
      }
      event "btnGetIP": Value Change {
        n255 = event-data() -> ()  [unwired: 1 in, 1 out]
        n256 = Enqueue Element(queue=w460, element="btnGetIP" ("元素"), error in (no error)=w459) -> (error out=w461:errorcluster)  [unwired: 1 in, 2 out]
      }
      event "btnGetPort": Value Change {
        n257 = event-data() -> ()  [unwired: 1 in, 1 out]
        n258 = Enqueue Element(queue=w464, element="btnGetPort" ("元素"), error in (no error)=w463) -> (error out=w465:errorcluster)  [unwired: 1 in, 2 out]
      }
      event "btnSetConst": Value Change {
        n259 = event-data() -> ()  [unwired: 1 in, 1 out]
        n260 = Enqueue Element(queue=w468, element="btnSetConst" ("元素"), error in (no error)=w467) -> (error out=w469:errorcluster)  [unwired: 1 in, 2 out]
      }
      event "btnSetSweep": Value Change {
        n261 = event-data() -> ()  [unwired: 1 in, 1 out]
        n262 = Enqueue Element(queue=w472, element="btnSetSweep" ("元素"), error in (no error)=w471) -> (error out=w473:errorcluster)  [unwired: 1 in, 2 out]
      }
      event "btnSetFreerun": Value Change {
        n263 = event-data() -> ()  [unwired: 1 in, 1 out]
        n264 = Enqueue Element(queue=w476, element="btnSetFreerun" ("元素"), error in (no error)=w475) -> (error out=w477:errorcluster)  [unwired: 1 in, 2 out]
      }
      event "btnStart": Value Change {
        n265 = event-data() -> ()  [unwired: 1 in, 1 out]
        n266 = Enqueue Element(queue=w480, element="btnStart" ("元素"), error in (no error)=w479) -> (error out=w481:errorcluster)  [unwired: 1 in, 2 out]
      }
      event "btnStatus": Value Change {
        n267 = event-data() -> ()  [unwired: 1 in, 1 out]
        n268 = Enqueue Element(queue=w484, element="btnStatus" ("元素"), error in (no error)=w483) -> (error out=w485:errorcluster)  [unwired: 1 in, 2 out]
      }
      event "btnStop": Value Change {
        n269 = event-data() -> ()  [unwired: 1 in, 1 out]
        n270 = Enqueue Element(queue=w488, element="btnStop" ("元素"), error in (no error)=w487) -> (error out=w489:errorcluster)  [unwired: 1 in, 2 out]
      }
      event "btnGetch": Value Change {
        n271 = event-data() -> ()  [unwired: 1 in, 1 out]
        n272 = Enqueue Element(queue=w492, element="btnGetch" ("元素"), error in (no error)=w491) -> (error out=w493:errorcluster)  [unwired: 1 in, 2 out]
      }
      event "btnGetSlot": Value Change {
        n273 = event-data() -> ()  [unwired: 1 in, 1 out]
        n274 = Enqueue Element(queue=w496, element="btnGetSlot" ("元素"), error in (no error)=w495) -> (error out=w497:errorcluster)  [unwired: 1 in, 2 out]
      }
      event "btnGetParameter": Value Change {
        n275 = event-data() -> ()  [unwired: 1 in, 1 out]
        n276 = Enqueue Element(queue=w500, element="btnGetParameter" ("元素"), error in (no error)=w499) -> (error out=w501:errorcluster)  [unwired: 1 in, 2 out]
      }
      event "btnVisa": Value Change {
        n277 = event-data() -> ()  [unwired: 1 in, 1 out]
        n278 = Enqueue Element(queue=w504, element="btnVisa" ("元素"), error in (no error)=w503) -> (error out=w505:errorcluster)  [unwired: 1 in, 2 out]
      }
      event "Communication": Value Change {
        n279 = event-data() -> ()  [unwired: 1 in, 1 out]
        n280 = Enqueue Element(queue=w508, element="Communication" ("元素"), error in (no error)=w507) -> (error out=w509:errorcluster)  [unwired: 1 in, 2 out]
      }
      event Panel Close {
        n281 = event-data() -> ()  [unwired: 1 in, 1 out]
      }
    }
    n282 = Unbundle By Name(w386) -> ("status"=w389:bool)
    n283 = Or(x=w389, y=w388) -> (x .or. y?=w387:bool)
  }
  n284 = Release Queue(queue=w1, error in (no error)=w5) -> ()  [unwired: 1 in, 3 out]
